vi "Sub Super Duper_10_19_12a_JW.vi"(0 "VISA resource name":refnum<visa-resource-name>="GPIB0::17::INSTR", 1 "Sample Properties:":T6 {"Date Created" format="%<%Y/%m/%d>T"}, 2 "TRF Cluster":T7={"Step 4"=-38.0, "# of Loops"=1.0, "Transfer 2"=FALSE, "Start 4"=-2.0, "Total Points 2"=2, "Start 3"=40.0, "Stop 2"=-40.0, "Step 3"=-1.0, "Loop Step"=0.0, "Integration Time 3"=0, "Loop Wait"=0.0, "First Step"=0.0} {"Loop Wait" format="%<%H:%M:%S>t"; "Integration Time 3" scale=0.0..2.0; "Step 3" format="%.2f"; "Stop 2" format="%.2f"; "Start 3" format="%.2f"; "Start 4" format="%.2f"; "Step 4" format="%.2f"}, 3 "TSP Cluster":T8={"Transport"=FALSE, "Start 2"=0.0, "Stop 3"=-60.0, "Step 2"=-1.0, "Start"=0.0, "Step"=-10.0, "Total Points"=7, "Integration Time"=0} {"Integration Time" scale=0.0..2.0; "Step" format="%.2f"; "Start" format="%.2f"; "Step 2" format="%.2f"; "Stop 3" format="%.2f"; "Start 2" format="%.2f"}, 4 "Compliance Cluster":T3={"Var1 sweep settings"={"sweep spacing (linear: 0)"=0, "sweep mode"=FALSE, "compliance (V)"=100.0, "compliance (A)"=0.001}, "Var1 sweep settings 2"={"sweep spacing (linear: 0)"=0, "sweep mode"=FALSE, "compliance (V)"=100.0, "compliance (A)"=0.001}, "Var2 step settings 2"={"compliance (A)"=0.001, "compliance (V)"=100.0}, "Var2 step settings"={"compliance (A)"=0.001, "compliance (V)"=100.0}} {"Var2 step settings"."compliance (V)" format="%.2f"; "Var2 step settings"."compliance (A)" format="%^.2e"; "Var2 step settings 2"."compliance (V)" format="%.2f"; "Var2 step settings 2"."compliance (A)" format="%^.2e"; "Var1 sweep settings 2"."compliance (A)" format="%^.2e"; "Var1 sweep settings 2"."compliance (V)" format="%.2f"; "Var1 sweep settings 2"."sweep spacing (linear: 0)" items=["linear", "log 10", "log 25", "log 50"]; "Var1 sweep settings"."compliance (A)" format="%^.2e"; "Var1 sweep settings"."compliance (V)" format="%.2f"; "Var1 sweep settings"."sweep spacing (linear: 0)" items=["linear", "log 10", "log 25", "log 50"]}, 5 "error in":errorcluster, 6 "Saved Folder:":path=path "C:/1DATA/2011", 7 "Wait Cluster":T2 {"Wait Time (s)" format="%.1g"; "Wait Countdown" format="%<%H:%M:%S%1u>t"}, 9 "Stop \nCountdown":bool, 11 "Loop Count":dbl) -> (8 "Status Indicator":bool, 10 "Vt Cluster":T1 {"Id Max" format="%.3g"; "Vt Max" format="%.3g"; "Vt Min" format="%.3g"; "Vt Ratio" format="%.3g"}, 12 "Gate Current Graph - Transport":cluster{"trace":dbl[], "trace":dbl[]}(graph), 13 "Gate Current Graph - Transfer":cluster{"trace":dbl[], "trace":dbl[]}(graph), 14 "VISA resource name out":refnum<visa-resource-name>, 15 "TRF Path":path, 16 "TSP Path":path, 17 "Graph Cluster":T4, 18 "Char Cluster":T5 {"Mobility-Lin" format="%#_4e"; "On/Off" format="%#_4e"; "Mobility-Sat" format="%#_4e"}, 19 "error out":errorcluster)   [LabVIEW 2011]
uses:
  <vilib>/Platform/TimedLoop/XDataNode/wakeup.ctl
  <vilib>/Platform/TimedLoop/XDataNode/XDNodeRunTimeDep.lvlib
  <vilib>/Platform/TimedLoop/XDataNode/nitl_modes.ctl
  <vilib>/Platform/TimedLoop/XDataNode/timing_clust.ctl
  <vilib>/Platform/TimedLoop/XDataNode/XDataNode.xnode
panel:
  # "Vg Sweep"
  # "Vd Step"
  # "Loops and Integration Time"
  # "Device Characteristics"
  # "Sample Properties:"
  # "%"
  # "nm"
  # "Device Properties:"
  # "um"
  # "um"
  # "Vg Step"
  # "Vd Step"
  # "Integration Time"
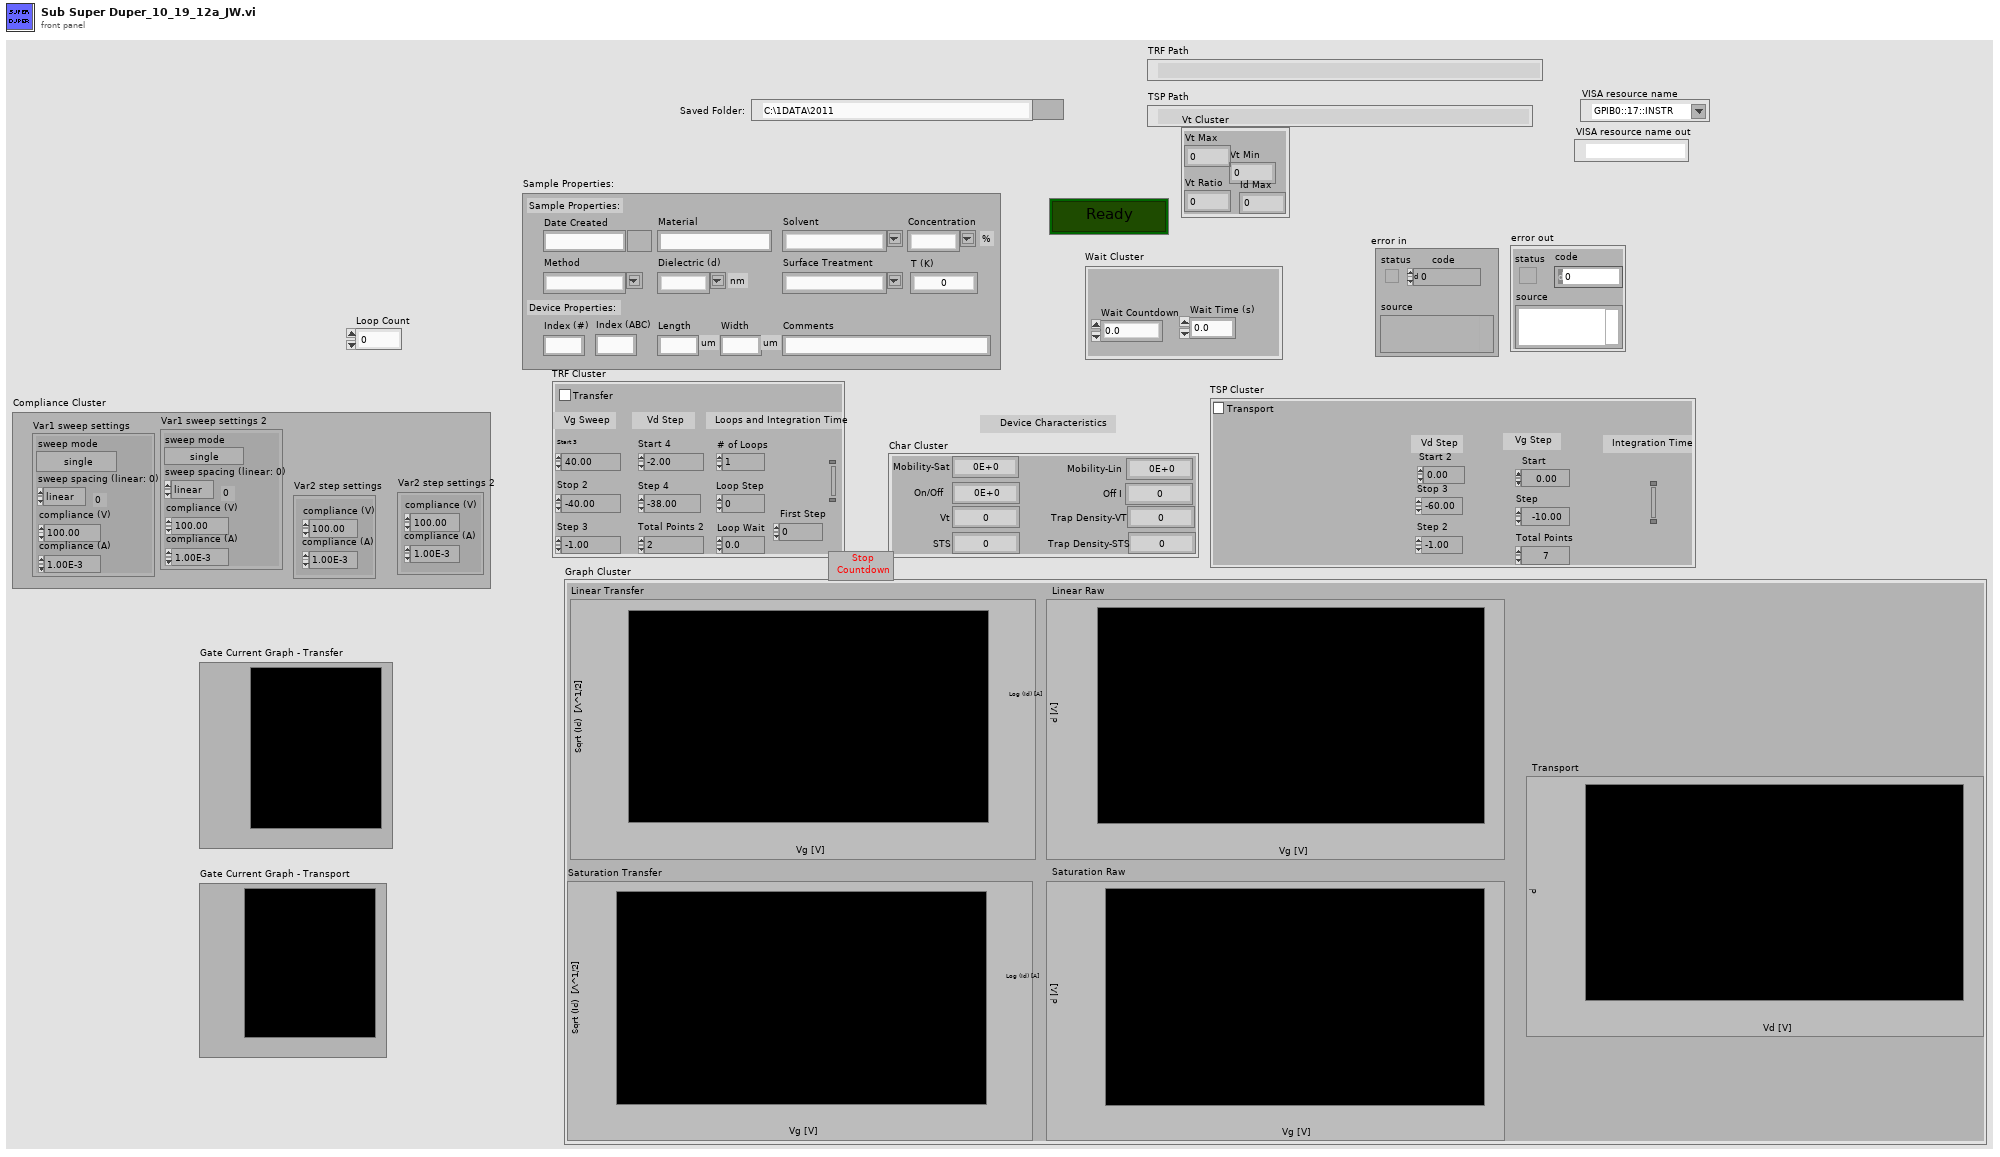
[diagram p1: front panel]
types:
  T1 = cluster{"Vt Max":i32, "Vt Min":i32, "Vt Ratio":i32, "Id Max":i32}
  T2 = cluster{"Wait Countdown":dbl, "Wait Time (s)":dbl}
  T3 = cluster{"Var1 sweep settings":cluster{"sweep spacing (linear: 0)":u16, "sweep mode":bool, "compliance (V)":dbl, "compliance (A)":dbl}, "Var1 sweep settings 2":cluster{"sweep spacing (linear: 0)":u16, "sweep mode":bool, "compliance (V)":dbl, "compliance (A)":dbl}, "Var2 step settings 2":cluster{"compliance (A)":dbl, "compliance (V)":dbl}, "Var2 step settings":cluster{"compliance (A)":dbl, "compliance (V)":dbl}}
  T4 = cluster{"Linear Transfer":cluster{dbl[], "trace":dbl[]}[], "Linear Raw":cluster{dbl[], dbl[]}[], "Saturation Transfer":cluster{dbl[], "trace":dbl[]}[], "Saturation Raw":cluster{dbl[], dbl[]}[], "Transport":cluster{dbl[], dbl[]}[]}
  T5 = cluster{"Mobility-Sat":dbl, "Mobility-Lin":dbl, "On/Off ":dbl, "Off I":dbl, "Vt":dbl, "STS":dbl, "Trap Density-VT":dbl, "Trap Density-STS":dbl}
  T6 = cluster{"Date Created":timestamp, "Material":string, "Solvent":string, "Concentration":string, "Method":string, "Dielectric (d)":string, "Index (#)":string, "Index (ABC)":string, "Length":string, "Width":string, "Surface Treatment":string, "Comments":string, "T (K)":dbl}
  T7 = cluster{"Step 4":dbl, "# of Loops":dbl, "Transfer 2":bool, "Start 4":dbl, "Total Points 2":u16, "Start 3":dbl, "Stop 2":dbl, "Step 3":dbl, "Loop Step":dbl, "Integration Time 3":u32, "Loop Wait":dbl, "First Step":dbl}
  T8 = cluster{"Transport":bool, "Start 2":dbl, "Stop 3":dbl, "Step 2":dbl, "Start":dbl, "Step":dbl, "Total Points":u16, "Integration Time":u32}
  T9 = typedef "XDNodeRunTimeDep.lvlib/timing_clust.ctl" = cluster{"Expected End [f-1]":u64, "Actual End [f-1]":u64, "Finished Late? [f-1]":bool, "Expected End [i-1]":u64, "Actual End [i-1]":u64, "Finished Late? [i-1]":bool, "Expected Start [i]":u64, "Actual Start [i]":u64, "Expected Start [f]":u64, "Actual Start [f]":u64, "Source Name":string, "Structure Name":string, "Period":i64, "Deadline":i64, "Offset":i64, "Start":i64, "Priority":i32, "Timeout":i32, "Mode":T10, "Wakeup Reason":T11, "Error":errorcluster, "Source Type":string, "Secondary Source Type":string, "Global End Time":u64, "Global Start Time":u64, "Frame Duration":u64, "Iteration Duration":u64, "Assigned CPU":i32, "I/O Scan Engine Mode":u32}
  T10 = typedef "XDNodeRunTimeDep.lvlib/nitl_modes.ctl" = enum32{"No Change", "Process missed periods, maintain original phase", "Discard missed periods, maintain original phase", "Process missed periods, ignore original phase", "Discard missed periods, ignore original phase"}
  T11 = typedef "XDNodeRunTimeDep.lvlib/wakeup.ctl" = enum32{"Normal", "Aborted", "Asynchronous wakeup", "Timing source error", "Timed loop error", "Timeout"}
  T12 = cluster{"sweep spacing (linear: 0)":u16, "sweep mode":bool, "compliance (V)":dbl, "compliance (A)":dbl}
  T13 = cluster{"compliance (A)":dbl, "compliance (V)":dbl}
  T14 = cluster{"Start 3":dbl, "Stop 2":dbl, "Step 3":dbl, "sweep spacing (linear: 0)":u16, "sweep mode":bool, "compliance (V)":dbl, "compliance (A)":dbl}
  T15 = cluster{"compliance (A)":dbl, "compliance (V)":dbl, "Start 4":dbl, "Total Points 2":u16, dbl}
  T16 = cluster{"Vt Max":i32, "Vt Min":i32, "Vt Ratio":i32, "Id Max":dbl}
  T17 = cluster{"Mobility-Sat":dbl, "Mobility-Lin":dbl, "On/Off Current":dbl, "Off I":dbl, "Vt":dbl, "STS":dbl, "Trap Density-VT":dbl, "Trap Density-STS":dbl}
  T18 = cluster{"Linear Sqrt":cluster{dbl[], "trace":dbl[]}[], "Linear Log":cluster{dbl[], "trace":dbl[]}[], "Linear Raw":cluster{dbl[], dbl[]}[], "Saturation Sqrt":cluster{dbl[], "trace":dbl[]}[], "Saturation Log":cluster{dbl[], "trace":dbl[]}[], "Saturation Raw":cluster{dbl[], "trace":dbl[]}[]}
  T19 = cluster{"Start 2":dbl, "Stop 3":dbl, "Step 2":dbl, "sweep spacing (linear: 0)":u16, "sweep mode":bool, "compliance (V)":dbl, "compliance (A)":dbl}
  T20 = cluster{"compliance (A)":dbl, "compliance (V)":dbl, "Start":dbl, "Total Points":u16, "Step":dbl}
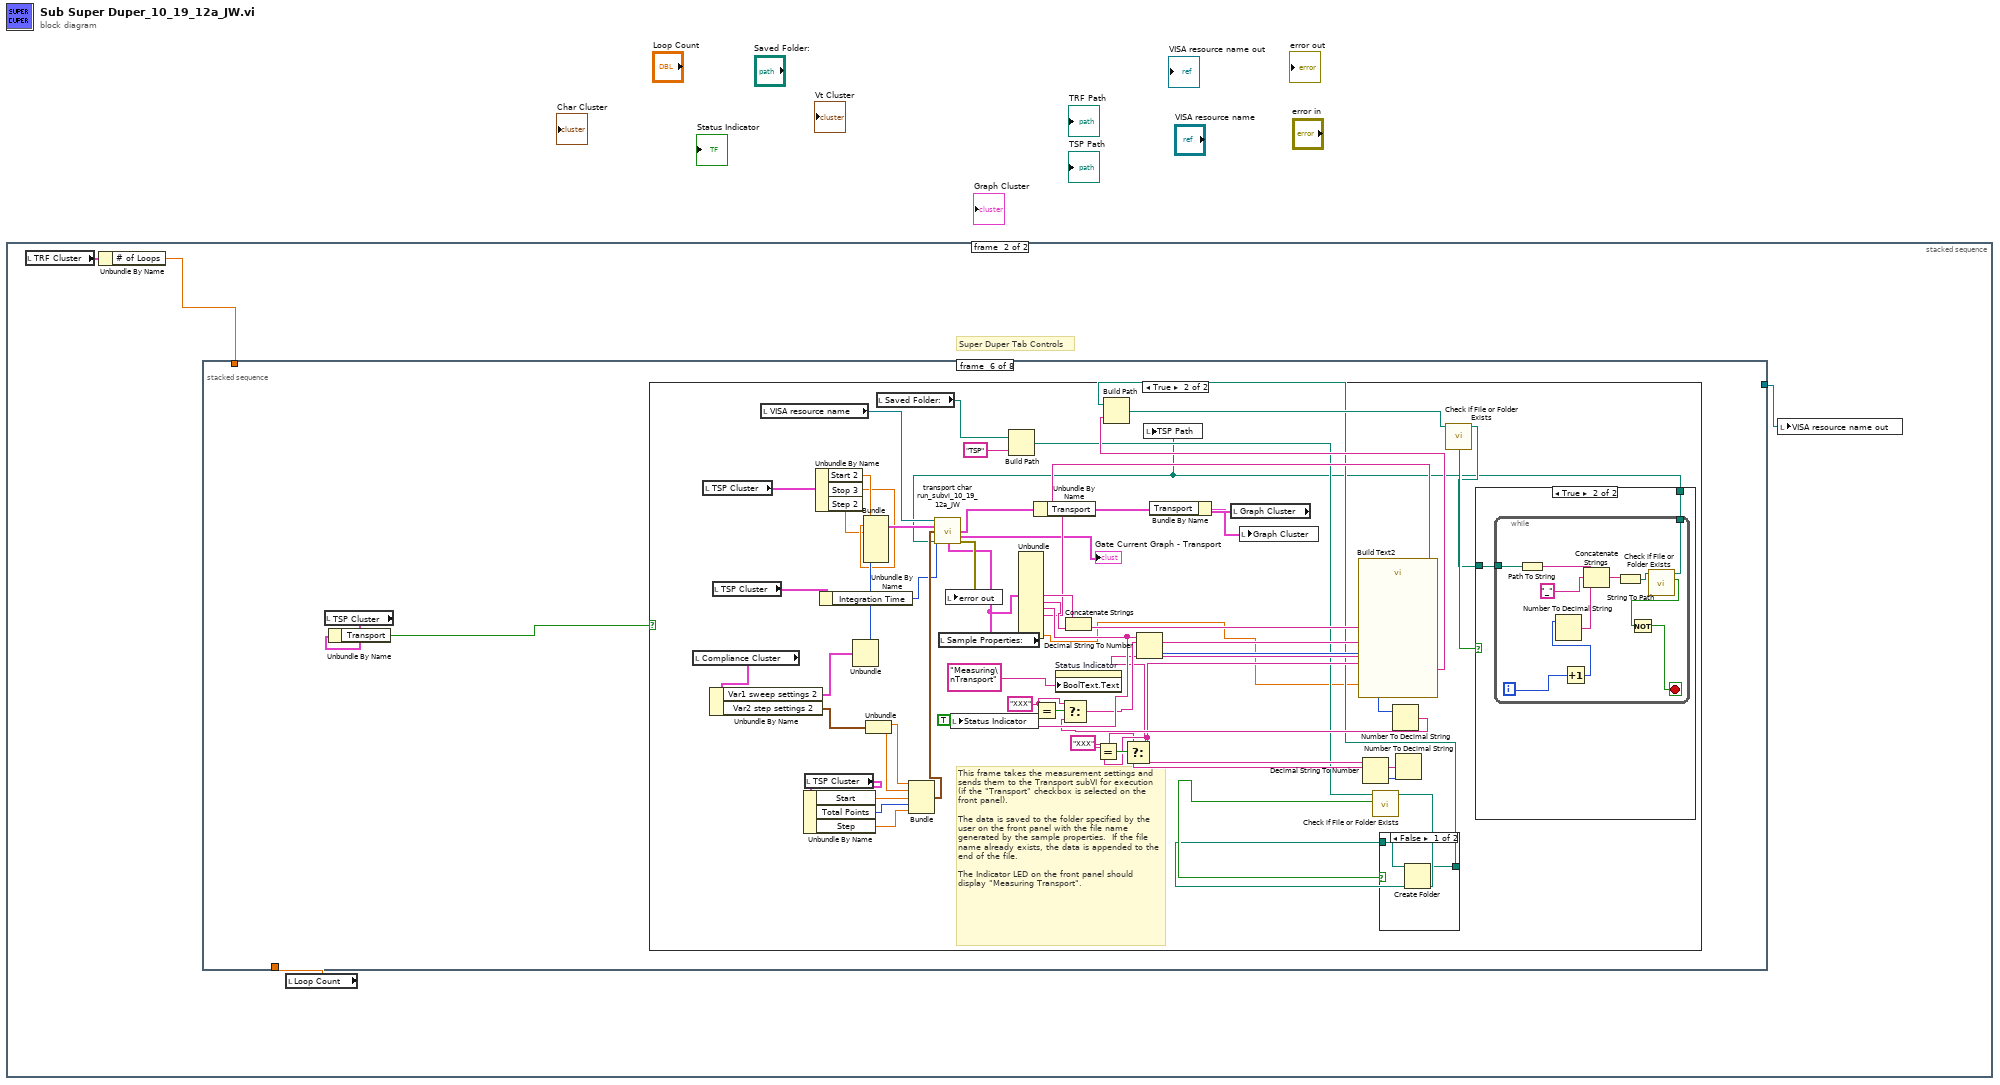
[diagram p0: block diagram]
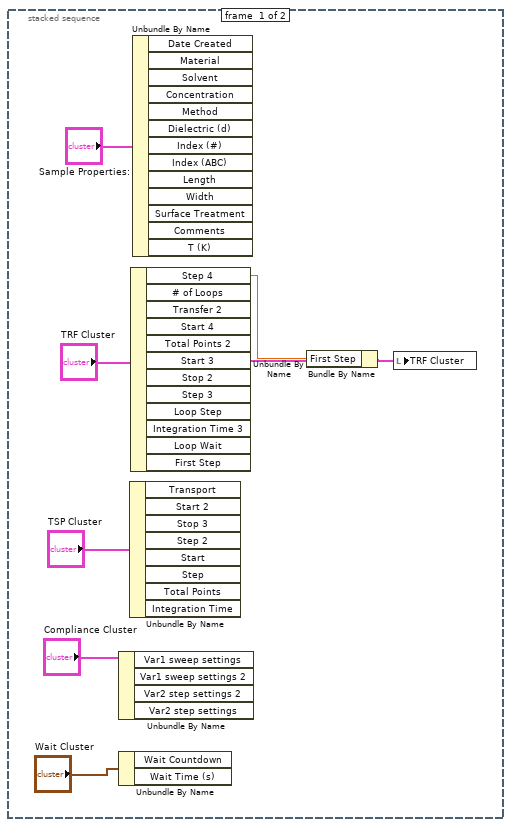
[diagram p2: hidden frame]
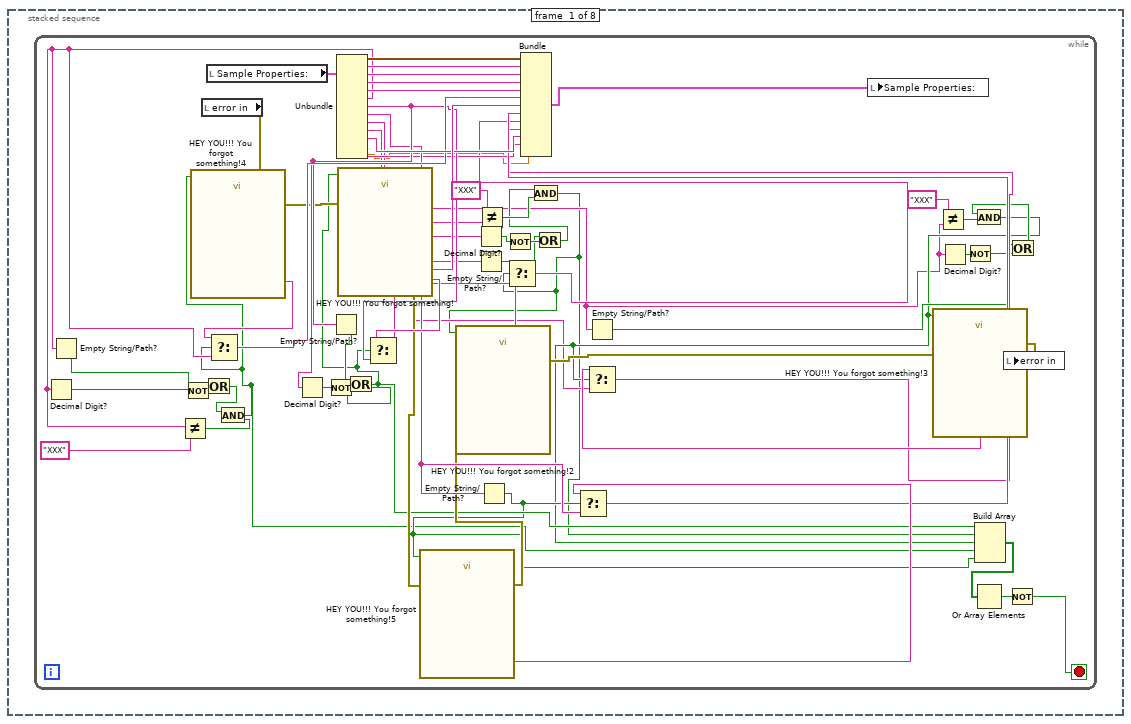
[diagram p3: hidden frame]
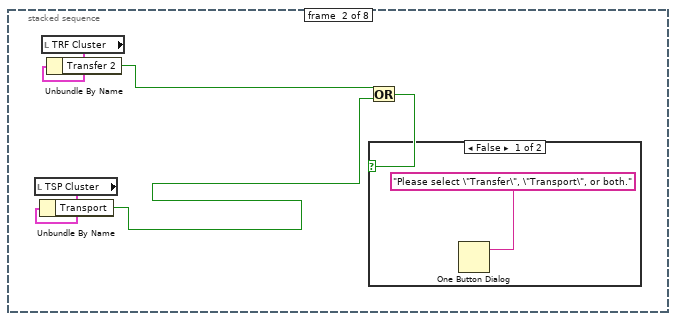
[diagram p4: hidden frame]
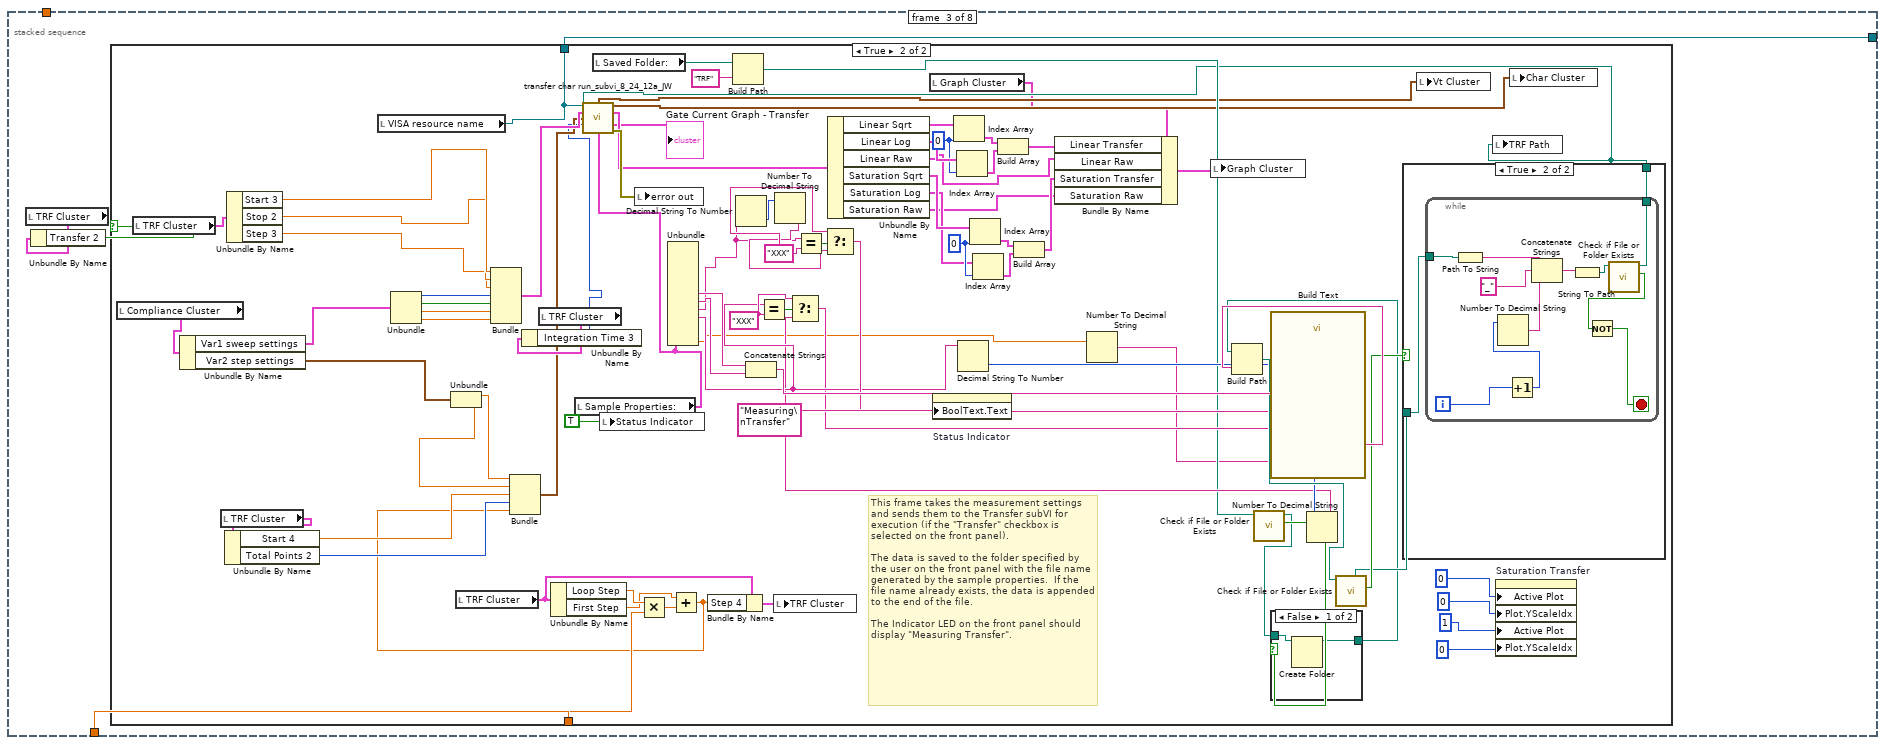
[diagram p6: hidden frame]
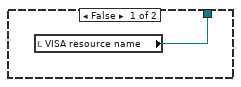
[diagram p7: hidden frame]
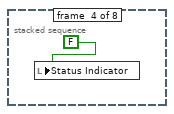
[diagram p10: hidden frame]
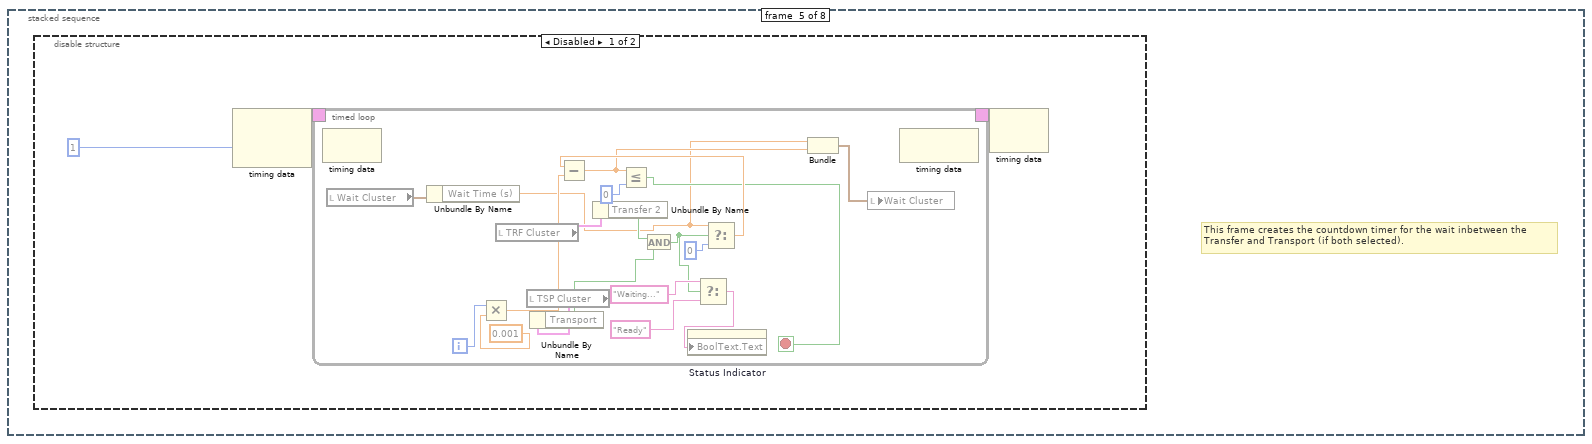
[diagram p11: hidden frame]
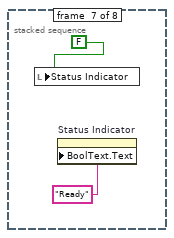
[diagram p16: hidden frame]
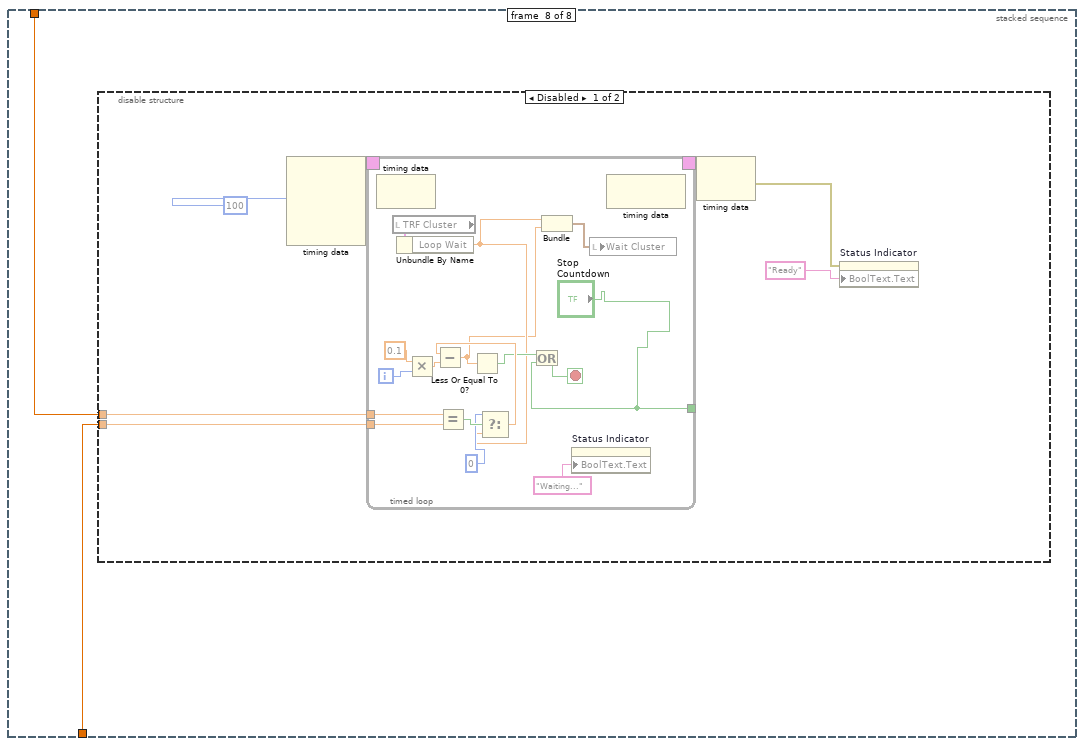
[diagram p17: hidden frame]
diagram:
  n1 = stacked-sequence {
    frame #0 {
      n2 = Unbundle By Name("Compliance Cluster") -> ()  [unwired: 4 out]
      n3 = Unbundle By Name("Wait Cluster") -> ()  [unwired: 2 out]
      n4 = Unbundle By Name("TSP Cluster") -> ()  [unwired: 8 out]
      n5 = Unbundle By Name("TRF Cluster") -> ("Step 4"=w7:dbl)  [unwired: 11 out]
      n6 = Unbundle By Name("Sample Properties:") -> ()  [unwired: 13 out]
      n7 = Bundle By Name(cluster="TRF Cluster", "First Step"=w7) -> (w5:T7)
      n8 = local write "TRF Cluster"(w5) -> ()
    }
    frame #1 {
      # "Super Duper Tab Controls"
      n9 = local read "TRF Cluster"() -> (w11:T7)
      n10 = Unbundle By Name(w11) -> ("# of Loops"=w10:dbl)
      n11 = local read "Loop Count"() -> (w8:dbl)
      n12 = stacked-sequence {
        tunnel: w8 -> [_ _ w81 _ _ _ _ w293]
        tunnel: w10 -> [_ _ _ _ _ _ _ w292]
        tunnel: [_ _ w78 _ _ _ _ _] -> w9
        frame #0 {
          n13 = while {
            stop <- w37 stop-if-true
            n14 = local read "error in"() -> (w43:errorcluster)
            n15 = local read "Sample Properties:"() -> (w66:T6)
            n16 = Unbundle(w66) -> ("Date Created"=w67:timestamp, "Material"=w68:string, "Solvent"=w69:string, "Concentration"=w70:string, "Method"=w71:string, "Dielectric (d)"=w26:string, "Index (#)"=w56:string, "Index (ABC)"=w53:string, "Length"=w21:string, "Width"=w14:string, "Surface Treatment"=w59:string, "Comments"=w51:string, "T (K)"=w12:dbl)
            n17 = Decimal Digit?(1:w26) -> (0:w34:bool)
            n18 = Empty String/Path?(string/path=w26) -> (empty?=w28:bool)
            n19 = Not Equal?(x=w26, y="XXX") -> (x != y?=w25:bool)
            n20 = Not(x=w34) -> (.not. x?=w31:bool)
            n21 = Or(x=w28, y=w31) -> (x .or. y?=w24:bool)
            n22 = And(x=w24, y=w25) -> (x .and. y?=w23:bool)
            n23 = call "HEY YOU!!! You forgot something!4"("Enable"=w23, "error in (no error)"=w43) -> ("Dielectric (d)"=w58:string, "error out"=w42:errorcluster)  [unwired: 15 in, 1 out]
            n24 = Select(t=w58, s=w23, f=w26) -> (s? t:f=w57:string)
            n25 = Decimal Digit?(1:w56) -> (0:w47:bool)
            n26 = Not(x=w47) -> (.not. x?=w46:bool)
            n27 = Empty String/Path?(string/path=w56) -> (empty?=w55:bool)
            n28 = Or(x=w55, y=w46) -> (x .or. y?=w41:bool)
            n29 = call "HEY YOU!!! You forgot something!"("Enable"=w41, "error in (no error)"=w42) -> ("Index (#)"=w65:string, "error out"=w45:errorcluster)  [unwired: 15 in, 1 out]
            n30 = Select(t=w65, s=w41, f=w56) -> (s? t:f=w62:string)
            n31 = Decimal Digit?(1:w21) -> (0:w36:bool)
            n32 = Empty String/Path?(string/path=w21) -> (empty?=w30:bool)
            n33 = Not Equal?(x="XXX", y=w21) -> (x != y?=w20:bool)
            n34 = Empty String/Path?(string/path=w53) -> (empty?=w40:bool)
            n35 = call "HEY YOU!!! You forgot something!5"("Enable"=w40, "error in (no error)"=w45) -> ("Index (ABC)"=w54:string, "error out"=w44:errorcluster)  [unwired: 15 in, 1 out]
            n36 = Not(x=w36) -> (.not. x?=w33:bool)
            n37 = Or(x=w30, y=w33) -> (x .or. y?=w19:bool)
            n38 = And(x=w19, y=w20) -> (x .and. y?=w13:bool)
            n39 = call "HEY YOU!!! You forgot something!2"("Enable"=w13, "error in (no error)"=w44) -> ("Length"=w64:string, "error out"=w61:errorcluster)  [unwired: 15 in, 1 out]
            n40 = Select(t=w64, s=w13, f=w21) -> (s? t:f=w50:string)
            n41 = Select(t=w54, s=w40, f=w53) -> (s? t:f=w52:string)
            n42 = Empty String/Path?(string/path=w14) -> (empty?=w29:bool)
            n43 = Not Equal?(x="XXX", y=w14) -> (x != y?=w18:bool)
            n44 = Decimal Digit?(1:w14) -> (0:w35:bool)
            n45 = Not(x=w35) -> (.not. x?=w32:bool)
            n46 = Or(x=w29, y=w32) -> (x .or. y?=w17:bool)
            n47 = And(x=w17, y=w18) -> (x .and. y?=w16:bool)
            n48 = call "HEY YOU!!! You forgot something!3"("Enable"=w16, "error in (no error)"=w61) -> ("Width"=w63:string, "error out"=w60:errorcluster)  [unwired: 15 in, 1 out]
            n49 = Select(t=w63, s=w16, f=w14) -> (s? t:f=w49:string)
            n50 = Bundle("Date Created"=w67, "Material"=w68, "Solvent"=w69, "Concentration"=w70, "Method"=w71, "Dielectric (d)"=w57, "Index (#)"=w62, "Index (ABC)"=w52, "Length"=w50, "Width"=w49, "Surface Treatment"=w59, "Comments"=w51, "T (K)"=w12) -> (w48:T6)  [unwired: 1 in]
            n51 = local write "Sample Properties:"(w48) -> ()
            n52 = Build Array(w41, w13, w16, w23, w40) -> (w39:bool[])
            n53 = Or Array Elements(Boolean array=w39) -> (logical OR=w38:bool)
            n54 = local write "error in"(w60) -> ()
            n55 = Not(x=w38) -> (.not. x?=w37:bool)
          }
        }
        frame #1 {
          n56 = local read "TSP Cluster"() -> (w73:T8)
          n57 = Unbundle By Name(w73) -> ("Transport"=w72:bool)
          n58 = local read "TRF Cluster"() -> (w75:T7)
          n59 = Unbundle By Name(w75) -> ("Transfer 2"=w74:bool)
          n60 = Or(x=w74, y=w72) -> (x .or. y?=w76:bool)
          n61 = case shown="False" w76 {
            frame False {
              n62 = One Button Dialog(message="Please select \"Transfer\", \"Transport\", or both.") -> ()  [unwired: 1 in, 1 out]
            }
            frame True {
            }
          }
        }
        frame #2 {
          n63 = local read "TRF Cluster"() -> (w79:T7)
          n64 = Unbundle By Name(w79) -> ("Transfer 2"=w80:bool)
          n65 = case shown="True" w80 {
            tunnel: w81 -> [_ w115]
            tunnel: [w82 w109] -> w78
            frame False {
              n66 = local read "VISA resource name"() -> (w82:refnum<visa-resource-name>)
            }
            frame True {
              w90 = 0
              w96 = 0
              w144 = "XXX"
              w148 = "XXX"
              # "This frame takes the measurement settings and sends them to the Transfer subVI for execution (if the \"Transfer\" checkbox is selected on the front panel).\n\nThe data is saved to the folder specified by the user on the front panel with the file name generated by the sample properties.  If the file name already exists, the data is appended to the end of the file.\n\nThe Indicator LED on the front panel should display \"Measuring Transfer\"."
              n67 = local read "Compliance Cluster"() -> (w121:T3)
              n68 = local read "TRF Cluster"() -> (w127:T7)
              n69 = Unbundle By Name(w121) -> ("Var1 sweep settings"=w119:T12, "Var2 step settings"=w120:T13)
              n70 = local read "TRF Cluster"() -> (w130:T7)
              n71 = Unbundle By Name(w130) -> ("Start 4"=w129:dbl, "Total Points 2"=w128:u16)
              n72 = Unbundle By Name(w127) -> ("Start 3"=w126:dbl, "Stop 2"=w125:dbl, "Step 3"=w124:dbl)
              n73 = local read "VISA resource name"() -> (w109:refnum<visa-resource-name>)
              n74 = Unbundle(w119) -> ("sweep spacing (linear: 0)"=w166:u16, "sweep mode"=w165:bool, "compliance (V)"=w164:dbl, "compliance (A)"=w163:dbl)
              n75 = Unbundle(w120) -> ("compliance (A)"=w162:dbl, "compliance (V)"=w161:dbl)
              n76 = local read "TRF Cluster"() -> (w110:T7)
              n77 = Bundle("Start 3"=w126, "Stop 2"=w125, "Step 3"=w124, "sweep spacing (linear: 0)"=w166, "sweep mode"=w165, "compliance (V)"=w164, "compliance (A)"=w163) -> (w108:T14)  [unwired: 1 in]
              n78 = local read "TRF Cluster"() -> (w123:T7)
              n79 = Unbundle By Name(w123) -> ("Integration Time 3"=w106:u32)
              n80 = Unbundle By Name(w110) -> ("Loop Step"=w113:dbl, "First Step"=w112:dbl)
              n81 = local read "Sample Properties:"() -> (w104:T6)
              n82 = local read "Saved Folder:"() -> (w122:path)
              n83 = local write "Status Indicator"(TRUE) -> ()
              n84 = Multiply(x=w113, y=w115) -> (x*y=w116:dbl)
              n85 = Unbundle(w104) -> ("Index (#)"=w157:string, "Index (ABC)"=w156:string, "Length"=w140:string, "Width"=w143:string, "T (K)"=w118:dbl)  [unwired: 8 out]
              n86 = Add(x=w112, y=w116) -> (x+y=w111:dbl)
              n87 = Bundle("compliance (A)"=w162, "compliance (V)"=w161, "Start 4"=w129, "Total Points 2"=w128, w111) -> (w107:T15)  [unwired: 1 in]
              n88 = Bundle By Name(cluster=w110, "Step 4"=w111) -> (w114:T7)
              n89 = Build Path(base path=w122, name or relative path="TRF") -> (appended path=w136:path)
              n90 = Decimal String To Number(string=w140) -> (number=w151:i32)  [unwired: 2 in, 1 out]
              n91 = Concatenate Strings(w157, w156) -> (w155:string)
              n92 = Equal?(x=w143, y=w144) -> (x = y?=w145:bool)
              n93 = local write "TRF Cluster"(w114) -> ()
              n94 = Number To Decimal String(number=w151) -> (decimal integer string=w147:string)  [unwired: 1 in]
              n95 = Equal?(x=w140, y=w148) -> (x = y?=w149:bool)
              n96 = Select(t=w148, s=w149, f=w147) -> (s? t:f=w146:string)
              n97 = local read "Graph Cluster"() -> (w99:T4)
              n98 = property on="Status Indicator" class="Bool (strict)"("BoolText.Text"="Measuring\nTransfer") -> ()  [unwired: 2 in, 2 out]
              n99 = Decimal String To Number(string=w143) -> (number=w150:i32)  [unwired: 2 in, 1 out]
              n100 = Number To Decimal String(number=w118) -> (decimal integer string=w117:string)  [unwired: 1 in]
              n101 = call <vilib>:"Check if File or Folder Exists.vi"("path"=w136) -> ("file or folder exists?"=w138:bool, "dup path"=w137:path)  [unwired: 8 in, 1 out]
              n102 = case shown="False" w138 {
                tunnel: w137 -> [w168 w169]
                tunnel: [w167 w169] -> w135
                frame False {
                  n103 = Create Folder(path (use dialog)=w168) -> (created path=w167:path)  [unwired: 2 in, 2 out]
                }
                frame True {
                }
              }
              n104 = Number To Decimal String(number=w150) -> (decimal integer string=w142:string)  [unwired: 1 in]
              n105 = Select(t=w144, s=w145, f=w142) -> (s? t:f=w141:string)
              n106 = call "Build Text"("T"=w117, "Index"=w155, "Length"=w146, "Width"=w141) -> ("Result"=w160:string)  [unwired: 10 in, 1 out]
              n107 = Build Path(base path=w135, name or relative path=w160) -> (appended path=w153:path)
              n108 = call <vilib>:"Check if File or Folder Exists.vi"("path"=w153) -> ("file or folder exists?"=w154:bool, "dup path"=w152:path)  [unwired: 8 in, 1 out]
              n109 = case shown="True" w154 {
                tunnel: w152 -> [w170 w172]
                tunnel: [w170 w171] -> w105
                frame False {
                }
                frame True {
                  n110 = while {
                    tunnel: w172 -> [w174]
                    tunnel: [w173] -> w171
                    i -> [w176]
                    stop <- w177 stop-if-true
                    n111 = Path To String(path=w174) -> (string=w183:string)
                    n112 = Increment(x=w176) -> (x+1=w175:i32)
                    n113 = Number To Decimal String(number=w175) -> (decimal integer string=w181:string)  [unwired: 1 in]
                    n114 = Concatenate Strings(w183, "_", w181) -> (w180:string)
                    n115 = String To Path(string=w180) -> (path=w179:path)
                    n116 = call <vilib>:"Check if File or Folder Exists.vi"("path"=w179) -> ("file or folder exists?"=w178:bool, "dup path"=w173:path)  [unwired: 8 in, 1 out]
                    n117 = Not(x=w178) -> (.not. x?=w177:bool)
                  }
                }
              }
              n118 = call "transfer char run_subvi_8_24_12a_JW.vi"("VISA session"=w109, "Var1 sweep settings"=w108, "Var2 step settings"=w107, "integration time"=w106, "Input Path"=w105, "Sample Properties:"=w104) -> ("Check Cluster"=w101:T16, "Output"=w102:T17, "Graph Cluster"=w100:T18, "Gate Current Graph"=→"Gate Current Graph - Transfer":cluster{"trace":dbl[], "trace":dbl[]}, "error?"=w103:errorcluster)  [unwired: 5 in]
              n119 = local write "error out"(w103) -> ()
              n120 = Unbundle By Name(w100) -> ("Linear Sqrt"=w98:cluster{dbl[], "trace":dbl[]}[], "Linear Log"=w97:cluster{dbl[], "trace":dbl[]}[], "Linear Raw"=w86:cluster{dbl[], dbl[]}[], "Saturation Sqrt"=w89:cluster{dbl[], "trace":dbl[]}[], "Saturation Log"=w88:cluster{dbl[], "trace":dbl[]}[], "Saturation Raw"=w85:cluster{dbl[], "trace":dbl[]}[])
              n121 = Index Array(array=w98, index=w96) -> (element=w95:cluster{dbl[], "trace":dbl[]})
              n122 = Index Array(array=w97, index=w96) -> (element=w94:cluster{dbl[], "trace":dbl[]})
              n123 = Index Array(array=w89, index=w90) -> (element=w91:cluster{dbl[], "trace":dbl[]})
              n124 = Index Array(array=w88, index=w90) -> (element=w92:cluster{dbl[], "trace":dbl[]})
              n125 = Build Array(w95, w94) -> (w93:cluster{dbl[], "trace":dbl[]}[])
              n126 = Build Array(w91, w92) -> (w87:cluster{dbl[], "trace":dbl[]}[])
              n127 = Bundle By Name(cluster=w99, "Linear Transfer"=w93, "Linear Raw"=w86, "Saturation Transfer"=w87, "Saturation Raw"=w85) -> (w84:T4)
              n128 = local write "Graph Cluster"(w84) -> ()
              n129 = local write "Vt Cluster"(w101) -> ()
              n130 = local write "TRF Path"(w105) -> ()
              n131 = property on="Saturation Transfer" class="XYGraph (strict)"("Active Plot"=0, "Plot.YScaleIdx"=0, "Active Plot"=1, "Plot.YScaleIdx"=0) -> ()  [unwired: 2 in, 2 out]
              n132 = local write "Char Cluster"(w102) -> ()
            }
          }
        }
        frame #3 {
          n133 = local write "Status Indicator"(FALSE) -> ()
        }
        frame #4 {
          # "This frame creates the countdown timer for the wait inbetween the\nTransfer and Transport (if both selected)."
          n134 = disable-structure shown="Disabled" {
            frame Disabled {
              n135 = node-c288(1) -> (w187:T9)  [unwired: 1 in]
              n136 = timed-loop {
                timing: w187 -> [_]
                timing-out: [_] -> w186
                i -> [w198]
                stop <- w199 stop-if-true
                n137 = node-c288() -> ()  [unwired: 1 in, 1 out]
                n138 = local read "Wait Cluster"() -> (w191:T2)
                n139 = Unbundle By Name(w191) -> ("Wait Time (s)"=w189:dbl)
                n140 = Multiply(x=w198, y=0.001) -> (x*y=w196:dbl)
                n141 = local read "TRF Cluster"() -> (w192:T7)
                n142 = local read "TSP Cluster"() -> (w193:T8)
                n143 = Unbundle By Name(w193) -> ("Transport"=w194:bool)
                n144 = Unbundle By Name(w192) -> ("Transfer 2"=w195:bool)
                n145 = And(x=w195, y=w194) -> (x .and. y?=w203:bool)
                n146 = Select(t="Waiting...", s=w203, f="Ready") -> (s? t:f=w205:string)
                n147 = property on="Status Indicator" class="Bool (strict)"("BoolText.Text"=w205) -> ()  [unwired: 2 in, 2 out]
                n148 = Select(t=w189, s=w203, f=0) -> (s? t:f=w201:dbl)
                n149 = Subtract(x=w201, y=w196) -> (x-y=w190:dbl)
                n150 = Less Or Equal?(x=w190, y=0) -> (x <= y?=w199:bool)
                n151 = Bundle("Wait Time (s)"=w189, w190) -> (w188:cluster{"Wait Time (s)":dbl, dbl})  [unwired: 1 in]
                n152 = local write "Wait Cluster"(w188) -> ()
                n153 = node-c288() -> ()  [unwired: 1 in, 1 out]
              }
              n154 = node-c288(w186) -> ()  [unwired: 1 out]
            }
            frame Enabled {
            }
          }
        }
        frame #5 {
          n155 = local read "TSP Cluster"() -> (w214:T8)
          n156 = Unbundle By Name(w214) -> ("Transport"=w213:bool)
          n157 = case shown="True" w213 {
            frame False {
            }
            frame True {
              w245 = "XXX"
              w249 = "XXX"
              # "This frame takes the measurement settings and sends them to the Transport subVI for execution (if the \"Transport\" checkbox is selected on the front panel).\n\nThe data is saved to the folder specified by the user on the front panel with the file name generated by the sample properties.  If the file name already exists, the data is appended to the end of the file.\n\nThe Indicator LED on the front panel should display \"Measuring Transport\"."
              n158 = local read "Compliance Cluster"() -> (w224:T3)
              n159 = local read "TSP Cluster"() -> (w236:T8)
              n160 = Unbundle By Name(w224) -> ("Var1 sweep settings 2"=w223:T12, "Var2 step settings 2"=w222:T13)
              n161 = local read "TSP Cluster"() -> (w229:T8)
              n162 = local read "VISA resource name"() -> (w226:refnum<visa-resource-name>)
              n163 = local read "TSP Cluster"() -> (w227:T8)
              n164 = Unbundle By Name(w227) -> ("Start"=w232:dbl, "Total Points"=w231:u16, "Step"=w230:dbl)
              n165 = Unbundle By Name(w236) -> ("Start 2"=w235:dbl, "Stop 3"=w234:dbl, "Step 2"=w233:dbl)
              n166 = Unbundle By Name(w229) -> ("Integration Time"=w228:u32)
              n167 = Unbundle(w223) -> ("sweep spacing (linear: 0)"=w272:u16, "sweep mode"=w271:bool, "compliance (V)"=w270:dbl, "compliance (A)"=w269:dbl)
              n168 = Bundle("Start 2"=w235, "Stop 3"=w234, "Step 2"=w233, "sweep spacing (linear: 0)"=w272, "sweep mode"=w271, "compliance (V)"=w270, "compliance (A)"=w269) -> (w268:T19)  [unwired: 1 in]
              n169 = Unbundle(w222) -> ("compliance (A)"=w267:dbl, "compliance (V)"=w266:dbl)
              n170 = local read "Saved Folder:"() -> (w225:path)
              n171 = Bundle("compliance (A)"=w267, "compliance (V)"=w266, "Start"=w232, "Total Points"=w231, "Step"=w230) -> (w265:T20)  [unwired: 1 in]
              n172 = local read "Sample Properties:"() -> (w261:T6)
              n173 = local write "Status Indicator"(TRUE) -> ()
              n174 = Build Path(base path=w225, name or relative path="TSP") -> (appended path=w238:path)
              n175 = Unbundle(w261) -> ("Index (#)"=w260:string, "Index (ABC)"=w259:string, "Length"=w250:string, "Width"=w246:string, "T (K)"=w220:dbl)  [unwired: 8 out]
              n176 = Equal?(x=w249, y=w250) -> (x = y?=w251:bool)
              n177 = property on="Status Indicator" class="Bool (strict)"("BoolText.Text"="Measuring\nTransport") -> ()  [unwired: 2 in, 2 out]
              n178 = Concatenate Strings(w260, w259) -> (w258:string)
              n179 = Equal?(x=w245, y=w246) -> (x = y?=w254:bool)
              n180 = Decimal String To Number(string=w250) -> (number=w253:i32)  [unwired: 2 in, 1 out]
              n181 = local read "Graph Cluster"() -> (w218:T4)
              n182 = Decimal String To Number(string=w246) -> (number=w252:i32)  [unwired: 2 in, 1 out]
              n183 = call <vilib>:"Check if File or Folder Exists.vi"("path"=w238) -> ("file or folder exists?"=w240:bool, "dup path"=w239:path)  [unwired: 8 in, 1 out]
              n184 = case shown="False" w240 {
                tunnel: w239 -> [w274 w275]
                tunnel: [w273 w275] -> w237
                frame False {
                  n185 = Create Folder(path (use dialog)=w274) -> (created path=w273:path)  [unwired: 2 in, 2 out]
                }
                frame True {
                }
              }
              n186 = Number To Decimal String(number=w253) -> (decimal integer string=w248:string)  [unwired: 1 in]
              n187 = Select(t=w249, s=w251, f=w248) -> (s? t:f=w247:string)
              n188 = Number To Decimal String(number=w252) -> (decimal integer string=w244:string)  [unwired: 1 in]
              n189 = Select(t=w245, s=w254, f=w244) -> (s? t:f=w243:string)
              n190 = call "Build Text2"("T"=w220, "Index"=w258, "Length"=w247, "Width"=w243) -> ("Result"=w242:string)  [unwired: 10 in, 1 out]
              n191 = Build Path(base path=w237, name or relative path=w242) -> (appended path=w255:path)
              n192 = call <vilib>:"Check if File or Folder Exists.vi"("path"=w255) -> ("file or folder exists?"=w257:bool, "dup path"=w256:path)  [unwired: 8 in, 1 out]
              n193 = case shown="True" w257 {
                tunnel: w256 -> [w276 w278]
                tunnel: [w276 w277] -> w221
                frame False {
                }
                frame True {
                  n194 = while {
                    tunnel: w278 -> [w280]
                    tunnel: [w279] -> w277
                    i -> [w282]
                    stop <- w283 stop-if-true
                    n195 = Path To String(path=w280) -> (string=w289:string)
                    n196 = Increment(x=w282) -> (x+1=w281:i32)
                    n197 = Number To Decimal String(number=w281) -> (decimal integer string=w287:string)  [unwired: 1 in]
                    n198 = Concatenate Strings(w289, "_", w287) -> (w286:string)
                    n199 = String To Path(string=w286) -> (path=w285:path)
                    n200 = call <vilib>:"Check if File or Folder Exists.vi"("path"=w285) -> ("file or folder exists?"=w284:bool, "dup path"=w279:path)  [unwired: 8 in, 1 out]
                    n201 = Not(x=w284) -> (.not. x?=w283:bool)
                  }
                }
              }
              n202 = call "transport char run_subvi_10_19_12a_JW.vi"("VISA session"=w226, "Var1 sweep settings"=w268, "Var2 step settings"=w265, "integration time"=w228, "Path"=w221, "Sample Properties:"=w261) -> ("Graph Cluster"=w219:cluster{"Transport":cluster{dbl[], dbl[]}[]}, "Gate Current Graph"=→"Gate Current Graph - Transport":cluster{"trace":dbl[], "trace":dbl[]}, "error?"=w264:errorcluster)  [unwired: 6 in, 1 out]
              n203 = local write "error out"(w264) -> ()
              n204 = Unbundle By Name(w219) -> ("Transport"=w216:cluster{dbl[], dbl[]}[])
              n205 = local write "TSP Path"(w221) -> ()
              n206 = Bundle By Name(cluster=w218, "Transport"=w216) -> (w217:T4)
              n207 = local write "Graph Cluster"(w217) -> ()
            }
          }
        }
        frame #6 {
          n208 = local write "Status Indicator"(FALSE) -> ()
          n209 = property on="Status Indicator" class="Bool (strict)"("BoolText.Text"="Ready") -> ()  [unwired: 2 in, 2 out]
        }
        frame #7 {
          n210 = disable-structure shown="Disabled" {
            disable-tunnel: w293 -> [w295 _]
            disable-tunnel: w292 -> [w294 _]
            frame Disabled {
              n211 = node-c288(100) -> (w300:T9)  [unwired: 3 in]
              n212 = timed-loop {
                timing: w300 -> [_]
                timing-out: [_] -> w299
                tunnel: w295 -> [w311]
                tunnel: w294 -> [w310]
                tunnel: ["Stop \nCountdown"] -> _
                i -> [w316]
                stop <- w306 stop-if-true
                n213 = node-c288() -> ()  [unwired: 1 in, 1 out]
                n214 = local read "TRF Cluster"() -> (w305:T7)
                n215 = Unbundle By Name(w305) -> ("Loop Wait"=w303:dbl)
                n216 = Multiply(x=0.1, y=w316) -> (x*y=w314:dbl)
                n217 = Equal?(x=w310, y=w311) -> (x = y?=w312:bool)
                n218 = Select(t=0, s=w312, f=w303) -> (s? t:f=w308:dbl)
                n219 = Subtract(x=w308, y=w314) -> (x-y=w302:dbl)
                n220 = Less Or Equal To 0?(x=w302) -> (x <= 0?=w307:bool)
                n221 = Or(x=w307, y="Stop \nCountdown") -> (x .or. y?=w306:bool)
                n222 = Bundle("Loop Wait"=w303, w302) -> (w304:cluster{"Loop Wait":dbl, dbl})  [unwired: 1 in]
                n223 = property on="Status Indicator" class="Bool (strict)"("BoolText.Text"="Waiting...") -> ()  [unwired: 2 in, 2 out]
                n224 = local write "Wait Cluster"(w304) -> ()
                n225 = node-c288() -> ()  [unwired: 1 in, 1 out]
              }
              n226 = node-c288(w299) -> (w296:errorcluster)
              n227 = property on="Status Indicator" class="Bool (strict)"(error in=w296, "BoolText.Text"="Ready") -> ()  [unwired: 1 in, 2 out]
            }
            frame Enabled {
            }
          }
        }
      }
      n228 = local write "VISA resource name out"(w9) -> ()
    }
  }
